vi "Send commands to hardware.vi"   [LabVIEW 2020]
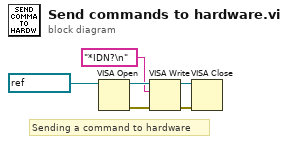
[diagram p0: block diagram]
diagram:
  # "Sending a command to hardware"
  n1 = VISA Open(VISA resource name=refnum<visa-resource-name> "COM3") -> (VISA resource name=w6:refnum<visa-resource-name>, error out=w5:errorcluster)  [unwired: 4 in]
  n2 = VISA Write(VISA resource name=w6, write buffer="*IDN?\n", error in (no error)=w5) -> (VISA resource name out=w4:refnum<visa-resource-name>, error out=w3:errorcluster)  [unwired: 1 out]
  n3 = VISA Close(VISA resource name=w4, error in (no error)=w3) -> ()  [unwired: 1 out]
